vi "Fdx Close Session (Port).vi"(8 "error in":errorcluster, 10 "InstrumentHandle_port in":u32, 11 "InstrumentHandle_board in":u32) -> (0 "error out":errorcluster)   [LabVIEW 2020, in "AIM664LV.lvlib"]
doc: "This function will close the reference to the board and the port in use."
uses:
  AIM664LV.lvlib
  _controls/hwEntry_actions.ctl
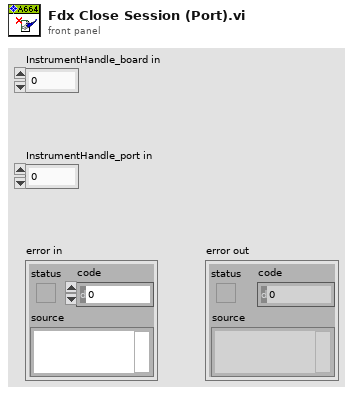
[diagram p1: front panel]
types:
  T1 = typedef "AIM664LV.lvlib/hwEntry_actions.ctl" = enum16{"Init Port", "Init Board", "Relase Port", "Release Board"}
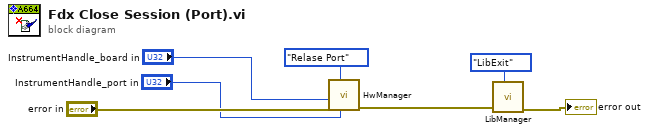
[diagram p0: block diagram]
diagram:
  n1 = call "HwManager.vi"("InstrumentHandle_port in"="InstrumentHandle_port in", "action (Init)"=hwEntry_actions."Relase Port" ("action"), "error in (no error)"="error in", "InstrumentHandle_board in"="InstrumentHandle_board in") -> ("error out"=w4:errorcluster)  [unwired: 3 in, 4 out]
  n2 = call "LibManager.vi"("action"=enum16{"LibInit", "LibExit"}."LibExit", "error in (no error)"=w4) -> ("error out"=→"error out":errorcluster)  [unwired: 7 in, 2 out]
